vi "Fit VI window to Largest Dec.vi"(4 "error in (no error)":errorcluster, 6 "border spacing (2 px)":i32=2, 7 "VI Ref (calling VI)":refnum<vi>) -> (0 "error out":errorcluster, 3 "dup VI Ref":refnum<vi>)   [LabVIEW 2020]
doc: "This utility will fit (resize and center) a VI (defined by the \"VI Ref\" input) about the largest decoration in that VI. It will add a border defined by border spacing in units of pixels. If there are no decorations found in the VI it is a no-op and will not produce an error. Unfortunately, this VI can not find locked decorations (yet)."
uses:
  <vilib>/Utility/miscctls.llb/LVPointTypeDef.ctl
panel:
  # "Fit VI window to Largest Decoration.vi\n\nFits a VI's front panel window to its largest decoration size.\n\nPlease visit http://www.OpenG.org to learn about the\nOpen Source LabVIEW software movement.\n\nNOTICE -- YOU MUST LEAVE THIS NOTICE IN PLACE.  PER THE TERMS OF THE LICENSE BELOW, YOU MAY SUBLICENSE THIS SOFTWARE \nIN ANY WAY THAT DOES NOT CONFLICT WITH THIS LICENSE.\n\n### BSD License (http://www.opensource.org/licenses/bsd-license.php) Begin ###\n \nCopyright (c) 2002, Jim Kring <jim@jimkring.com>\nCopyright (c) 2002, Cal-Bay Systems, Inc. <info@calbay.com>\n\nAll rights reserved.\n\nRedistribution and use in source and binary forms, with or without modification, are permitted provided that the following conditions are met:\n\n    * Redistributions of source code must retain the above copyright notice, this list of conditions and the following disclaimer.\n    * Redistributions in binary form must reproduce the above copyright notice, this list of conditions and the following disclaimer in the \n       documentation and/or other materials provided with the distribution.\n    * Neither the name of SciWare, James Kring, Inc., nor the names of its contributors may be used to endorse or promote products derived \n       from this software without specific prior written permission.\n\nTHIS SOFTWARE IS PROVIDED BY THE COPYRIGHT HOLDERS AND CONTRIBUTORS \"AS IS\" AND ANY EXPRESS OR IMPLIED WARRANTIES, \nINCLUDING, BUT NOT LIMITED TO, THE IMPLIED WARRANTIES OF MERCHANTABILITY AND FITNESS FOR A PARTICULAR PURPOSE ARE \nDISCLAIMED. IN NO EVENT SHALL THE COPYRIGHT OWNER OR CONTRIBUTORS BE LIABLE FOR ANY DIRECT, INDIRECT, INCIDENTAL,\n SPECIAL, EXEMPLARY, OR CONSEQUENTIAL DAMAGES (INCLUDING, BUT NOT LIMITED TO, PROCUREMENT OF SUBSTITUTE GOODS OR \nSERVICES; LOSS OF USE, DATA, OR PROFITS; OR BUSINESS INTERRUPTION) HOWEVER CAUSED AND ON ANY THEORY OF LIABILITY, \nWHETHER IN CONTRACT, STRICT LIABILITY, OR TORT (INCLUDING NEGLIGENCE OR OTHERWISE) ARISING IN ANY WAY OUT OF THE USE \nOF THIS SOFTWARE, EVEN IF ADVISED OF THE POSSIBILITY OF SUCH DAMAGE.\n\n### BSD License End ###"
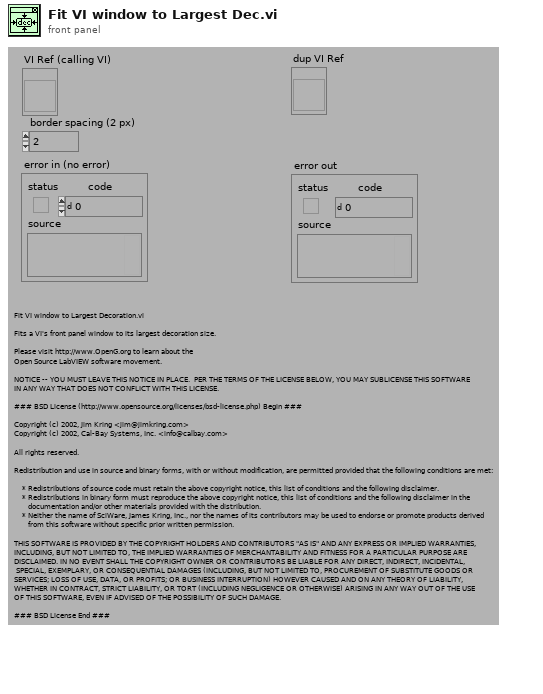
[diagram p1: front panel]
types:
  T1 = typedef "LVPointTypeDef.ctl" = cluster{"Horizontal":i16, "Vertical":i16}
  T2 = typedef "LVRectTypeDef.ctl" = cluster{"Left":i16, "Top":i16, "Right":i16, "Bottom":i16}
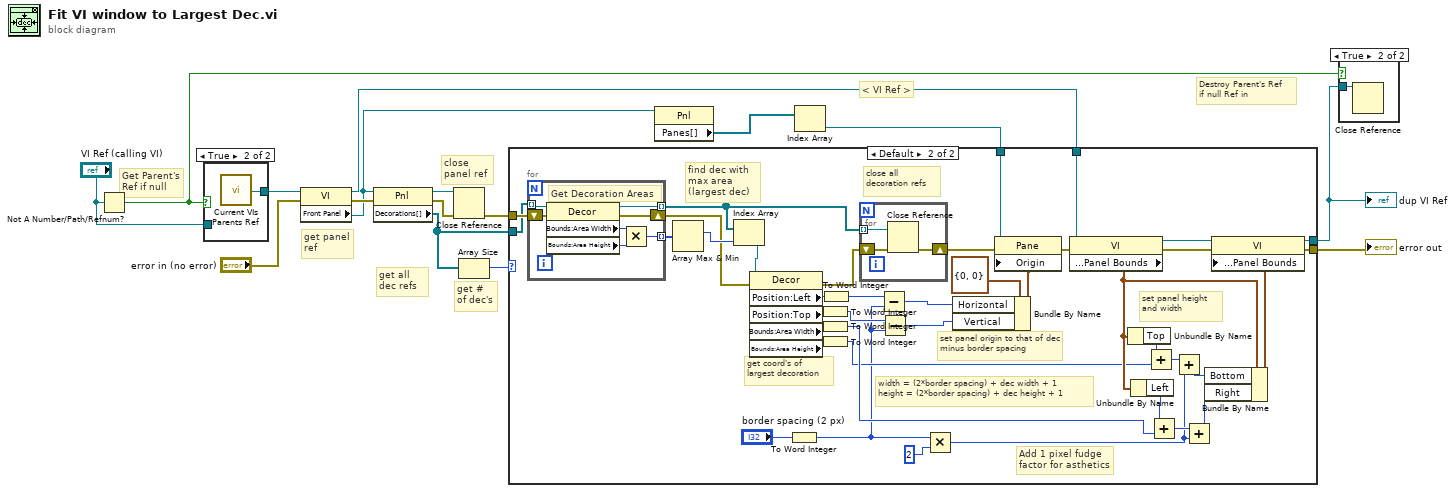
[diagram p0: block diagram]
diagram:
  # "Destroy Parent's Ref\nif null Ref in"
  # "Get Parent's\nRef if null"
  # "get # of dec's"
  # "get panel ref"
  # "get all dec refs"
  # "close panel ref"
  # "< VI Ref >"
  n1 = Not A Number/Path/Refnum?(number/path/refnum="VI Ref (calling VI)") -> (NaN/Path/Refnum?=w6:bool)
  n2 = case shown="True" w6 {
    tunnel: [w17 w18] -> w7
    tunnel: "VI Ref (calling VI)" -> [w17 _]
    frame False {
    }
    frame True {
      n3 = call "Current VIs Parents Ref.vi"() -> ("Calling VI's reference"=w18:refnum<vi>)  [unwired: 2 in]
    }
  }
  n4 = property on="Property Node" class="VI"(reference=w7, error in="error in (no error)") -> (reference out=w2:refnum<vi>, error out=w15:errorcluster, "Front Panel"=w3:refnum<vi>)
  n5 = property on="Property Node" class="Pnl"(reference=w3, error in=w15) -> (reference out=w16:refnum<vi>, error out=w14:errorcluster, "Decorations[]"=w10:refnum<vi>[])
  n6 = Close Reference(reference=w16, error in (no error)=w14) -> (error out=w12:errorcluster)
  n7 = Array Size(array=w10) -> (size(s)=w9:i32)
  n8 = property on="Property Node" class="Pnl"(reference=w3) -> ("Panes[]"=w4:refnum<vi>[])  [unwired: 1 in, 2 out]
  n9 = Index Array(array=w4) -> (element=w1:refnum<vi>)  [unwired: 1 in]
  n10 = case shown="Default" w9 {
    tunnel: w2 -> [w20 w24]
    tunnel: w12 -> [w19 w45]
    tunnel: [w19 w33] -> w11
    tunnel: [w20 w32] -> w5
    tunnel: w10 -> [_ w31]
    tunnel: w1 -> [_ w23]
    frame 0 {
      # "do nothing if no decorations"
    }
    frame Default {
      # "width = (2*border spacing) + dec width + 1\nheight = (2*border spacing) + dec height + 1"
      # "set panel height and width"
      # "set panel origin to that of dec minus border spacing"
      # "close all  decoration refs"
      # "get coord's of largest decoration"
      # "Add 1 pixel fudge factor for asthetics"
      # "find dec with max area (largest dec)"
      n11 = for {
        tunnel: w31 -> [w67] mode=indexing
        tunnel: [w64] -> w44 mode=indexing
        shift-right: [w62] -> w40
        shift-left: w45 -> [w63]
        tunnel: [w61] -> w42 mode=indexing
        # "Get Decoration Areas"
        n12 = property class="Decor"(reference=w67, error in=w63) -> (reference out=w61:refnum<vi>, error out=w62:errorcluster, "Bounds:Area Width"=w66:u32, "Bounds:Area Height"=w65:u32)
        n13 = Multiply(x=w66, y=w65) -> (x*y=w64:u32)
      }
      n14 = Array Max & Min(array=w44) -> (max index (indices)=w43:i32)  [unwired: 3 out]
      n15 = Index Array(array=w42, index=w43) -> (element=w41:refnum<vi>)
      n16 = property class="Decor"(reference=w41, error in=w40) -> (error out=w39:errorcluster, "Position:Left"=w46:i32, "Position:Top"=w49:i32, "Bounds:Area Width"=w54:u32, "Bounds:Area Height"=w52:u32)  [unwired: 1 out]
      n17 = To Word Integer(number="border spacing (2 px)") -> (16bit integer=w25:i16)
      n18 = To Word Integer(number=w49) -> (16bit integer=w26:i16)
      n19 = To Word Integer(number=w54) -> (16bit integer=w29:i16)
      n20 = To Word Integer(number=w52) -> (16bit integer=w28:i16)
      n21 = To Word Integer(number=w46) -> (16bit integer=w27:i16)
      n22 = for {
        tunnel: w42 -> [w70] mode=indexing
        shift-right: [w68] -> w36
        shift-left: w39 -> [w69]
        n23 = Close Reference(reference=w70, error in (no error)=w69) -> (error out=w68:errorcluster)
      }
      n24 = Subtract(x=w27, y=w25) -> (x-y=w47:i16)
      n25 = Subtract(x=w26, y=w25) -> (x-y=w48:i16)
      n26 = Multiply(x=w25, y=i16 2) -> (x*y=w30:i16)
      n27 = Bundle By Name(cluster=T1 {"Horizontal"=0, "Vertical"=0} ("Origin"), "Horizontal"=w47, "Vertical"=w48) -> (w21:T1)
      n28 = property on="Property Node" class="Pane"(reference=w23, error in=w36, "Origin"=w21) -> (error out=w35:errorcluster)  [unwired: 1 out]
      n29 = property on="Property Node" class="VI"(reference=w24, error in=w35) -> (reference out=w60:refnum<vi>, error out=w34:errorcluster, "Front Panel Window:Panel Bounds"=w50:T2)
      n30 = Unbundle By Name(w50) -> ("Top"=w51:i16)
      n31 = Unbundle By Name(w50) -> ("Left"=w53:i16)
      n32 = Add(x=w51, y=w28) -> (x+y=w58:i16)
      n33 = Add(x=w53, y=w29) -> (x+y=w56:i16)
      n34 = Add(x=w58, y=w30) -> (x+y=w59:i16)
      n35 = Add(x=w56, y=w30) -> (x+y=w57:i16)
      n36 = Bundle By Name(cluster=w50, "Bottom"=w59, "Right"=w57) -> (w55:T2)
      n37 = property on="Property Node" class="VI"(reference=w60, error in=w34, "Front Panel Window:Panel Bounds"=w55) -> (reference out=w32:refnum<vi>, error out=w33:errorcluster)
    }
  }
  "error out" <- w11
  "dup VI Ref" <- w5
  n38 = case shown="True" w6 {
    tunnel: w5 -> [_ w71]
    frame False {
    }
    frame True {
      n39 = Close Reference(reference=w71) -> ()  [unwired: 1 in, 1 out]
    }
  }
